vi "Execute.vi"(8 "error in":errorcluster, 11 "Set O2 Valve STEP in":refnum<class "O2 Valve STEP.lvclass">) -> (0 "error out":errorcluster, 1 "Next Step?":bool, 2 "MSG":string, 3 "Set O2 Valve STEP out":refnum<class "O2 Valve STEP.lvclass">)   [LabVIEW 2014, in "O2 Valve STEP.lvclass"]
uses:
  O2 Valve STEP.lvclass
  <vilib>/ActorFramework/Message Enqueuer/Message Enqueuer.lvclass
  Controller/Messages/O3 Valve MSG/O3 Valve MSG.lvclass
  reusable/Sequence/STEPS/STEP.lvclass/STEP.ctl
  Controller/Messages/Update Switch State MSG/Update Switch MSG.lvclass/Update Switch MSG.ctl
  <vilib>/ActorFramework/Message Enqueuer/Message Enqueuer.lvclass/Message Enqueuer.ctl
  reusable/Sequence/STEPS/Read Obj.vi
  Controller/Messages/Update Switch State MSG/Write SwitchState.vi
  <vilib>/ActorFramework/Message Priority Queue/Priority Enqueue.vi
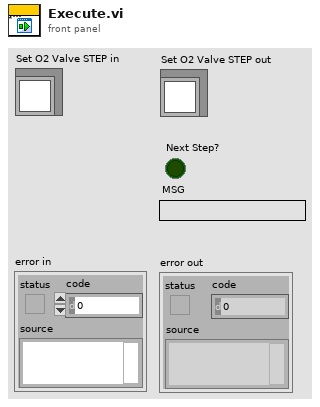
[diagram p1: front panel]
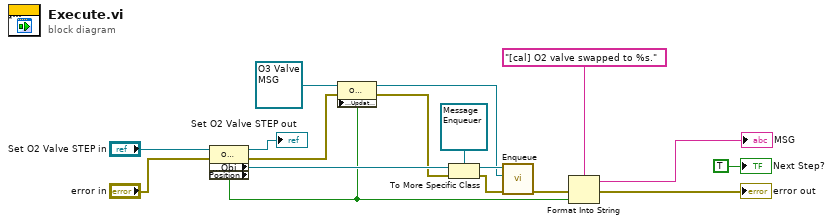
[diagram p0: block diagram]
diagram:
  n1 = property class="O2 Valve"(reference="Set O2 Valve STEP in", error in="error in") -> (reference out=→"Set O2 Valve STEP out":refnum<class "O2 Valve STEP.lvclass">, error out=w2:errorcluster, "Accessors:Obj"=w17:refnum<class>, "Position"=w5:bool)
  n2 = property class="O3 Valve"(reference=refnum<class "O3 Valve MSG.lvclass"> refnum ("Controller:O3 Valve"), error in=w2, "Accessors:UpdateSw"=w5) -> (reference out=w4:refnum<class "O3 Valve MSG.lvclass">, error out=w1:errorcluster)
  n3 = To More Specific Class(target class=refnum<class "Message Enqueuer.lvclass"> refnum ("Message Enqueuer in"), reference=w17, error in=w1) -> (specific class reference=w14:refnum<class "Message Enqueuer.lvclass">, error out=w15:errorcluster)
  n4 = call <vilib>:"Enqueue.vi"("error in (no error)"=w15, "Message"=w4, "Message Enqueuer in"=w14) -> ("error out"=w12:errorcluster)  [unwired: 7 in, 1 out]
  n5 = Format Into String(format string="[cal] O2 valve swapped to %s.", error in=w12, w5) -> (resulting string=→"MSG":string, error out=→"error out":errorcluster)  [unwired: 1 in]
  "Next Step?" <- TRUE ("Next Step?")
